vi "Lr5.vi"() -> ()   [LabVIEW 2012]
panel:
  in  "Cluster":T1 {"Noise" items=["Periodic Random", "Uniform white", "Gaussian white"]; "Sine frequency" scale=0.1..1.0; "Noise amplitude" scale=0.0..3.0; "Signal amplitude" scale=1.0..10.0; "Frequency" scale=0.1..100.0}
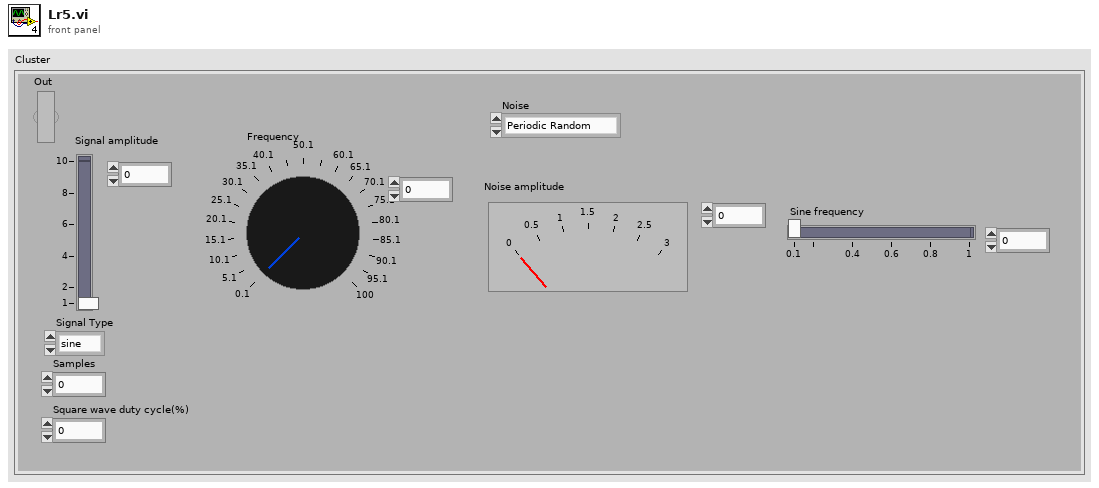
[diagram p1: front panel]
types:
  T1 = cluster{"Frequency":dbl, "Signal amplitude":dbl, "Square wave duty cycle(%)":dbl, "Signal Type":enum16{"sine", "square"}, "Noise amplitude":dbl, "Sine frequency":dbl, "Noise":u16, "Samples":i32, "Out":bool}
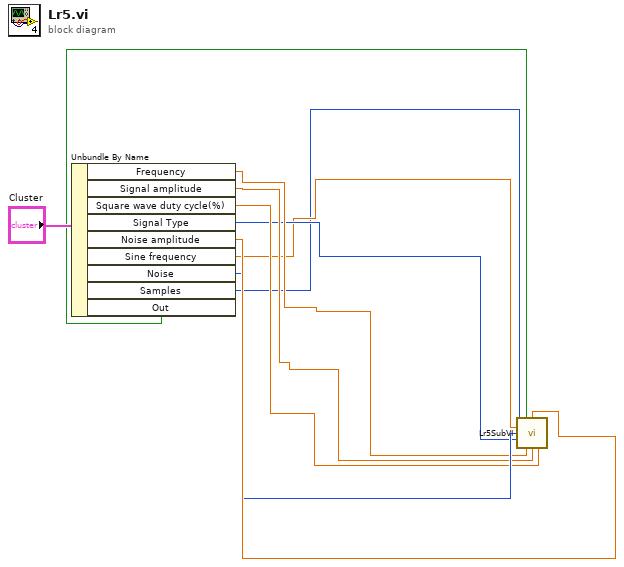
[diagram p0: block diagram]
diagram:
  n1 = Unbundle By Name("Cluster") -> ("Frequency"=w5:dbl, "Signal amplitude"=w6:dbl, "Square wave duty cycle(%)"=w7:dbl, "Signal Type"=w4:enum16{"sine", "square"}, "Noise amplitude"=w9:dbl, "Sine frequency"=w3:dbl, "Noise"=w8:u16, "Samples"=w2:i32, "Out"=w1:bool)
  n2 = call "Lr5SubVI.vi"("Samples"=w2, "Out"=w1, "Noise amplitude"=w9, "Sine frequency"=w3, "Noise"=w8, "Signal Type"=w4, "Frequency"=w5, "Signal amplitude"=w6, "Square wave duty cycle(%)"=w7) -> ()  [unwired: 7 in]
